vi "Set Property - Create Direction Folder.vi"(8 "error in":errorcluster, 9 "create Tx/Rx folders for subaddresses?":bool, 11 "custom device":T1 format="%.0x") -> (0 "error out":errorcluster, 3 "custom device out":T1 format="%.0x")   [LabVIEW 2023, in "Ballard MIL-STD-1553 Scripting.lvlib"]
uses:
  Ballard MIL-STD-1553 Scripting.lvlib
  <vilib>/NI VeriStand/Custom Device API/Custom Device Item Ref.ctl
  Constants.vi
  <vilib>/NI VeriStand/Custom Device API/Set Item Property (Boolean).vi
  <vilib>/NI VeriStand/Custom Device API/Custom Device API.lvlib
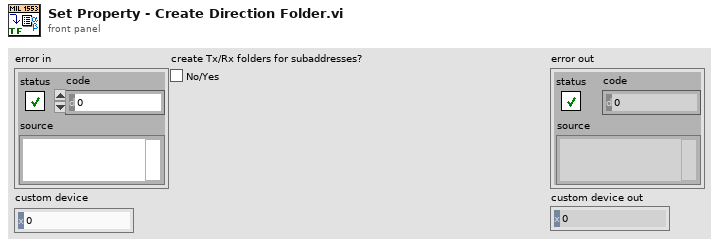
[diagram p1: front panel]
types:
  T1 = typedef "Custom Device API.lvlib/Custom Device Item Ref.ctl" = u64
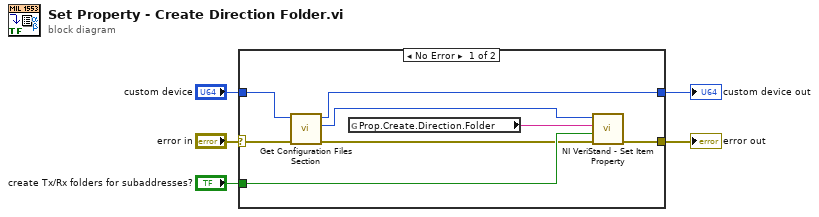
[diagram p0: block diagram]
diagram:
  n1 = case shown="No Error" "error in" {
    selector: "error in" -> [w11 w15]
    tunnel: "custom device" -> [w7 w14]
    tunnel: [w13 w15] -> w4
    tunnel: [w8 w14] -> w2
    tunnel: "create Tx/Rx folders for subaddresses?" -> [w12 _]
    frame No Error {
      n2 = call "Get Configuration Files Section.vi"("error in"=w11, "custom device in"=w7) -> ("error out"=w10:errorcluster, "configuration files section"=w9:T1, "custom device out"=w8:T1)  [unwired: 6 in, 1 out]
      n3 = global read "Constants.vi" "Prop.Create.Direction.Folder"() -> (w6:string)
      n4 = call-poly <vilib>:"NI VeriStand - Set Item Property.vi"("error in (no error)"=w10, "Value"=w12, "Property Name"=w6, "Item Ref in"=w9) -> ("error out"=w13:errorcluster)  [unwired: 5 in, 2 out]
    }
    frame Error {
    }
  }
  "error out" <- w4
  "custom device out" <- w2
